vi "Module Loop.vi"(8 "error in (no error)":errorcluster, 11 "DAQmxDO in":refnum<class "DAQmxDO.lvclass">) -> (0 "error out":errorcluster, 3 "DAQmxDO out":refnum<class "DAQmxDO.lvclass">)   [LabVIEW 2023, in "VolatusDAQ.lvlib" / "DAQmxDO.lvclass"]
uses:
  DAQmxDO.lvclass
  DAQmxDO.lvclass/DAQmxDO.ctl
  Volatus/Module/Module.lvclass
  lv-vecto/Vecto/Group DBL/Group DBL.lvclass
  VolatusData/Scaling/Scaling.lvclass
  lv-vecto/Vecto/Group/Group.lvclass
  lv-vecto/Vecto/Vecto.lvlib
  <vilib>/DAQmx/write.llb/DAQmx Write (Digital 1D Bool NChan 1Samp 1Line).vi
  C:/dev/volatus/mts-volatus-super/libs/lv-volatus/Volatus/Module/Module.lvclass
  C:/dev/volatus/mts-volatus-super/libs/lv-volatus/VolatusDAQ/DAQmxDO/DAQmxDO.lvclass
  C:/dev/volatus/mts-volatus-super/libs/lv-vecto/Vecto/Group/Group.lvclass
  C:/dev/volatus/mts-volatus-super/libs/lv-vecto/Vecto/Group DBL/Group DBL.lvclass
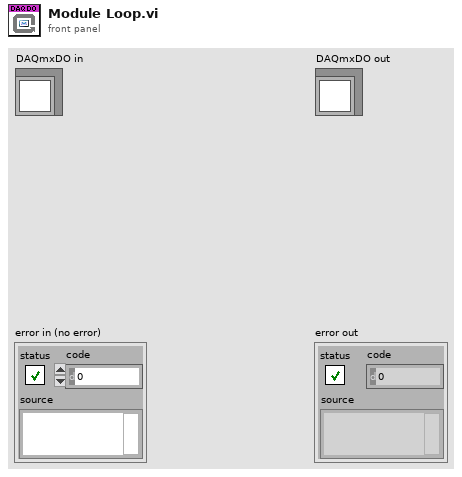
[diagram p1: front panel]
types:
  T1 = enum32{"Invalid", "Standard", "Closed", "Hidden", "Minimized", "Maximized"}
  T2 = typedef "CmdDigitalMultiple.lvlib/Data.ctl" = cluster{"values":T3[]}
  T3 = typedef "CmdDigital.lvlib/Data.ctl" = cluster{"channel":string, "value":bool}
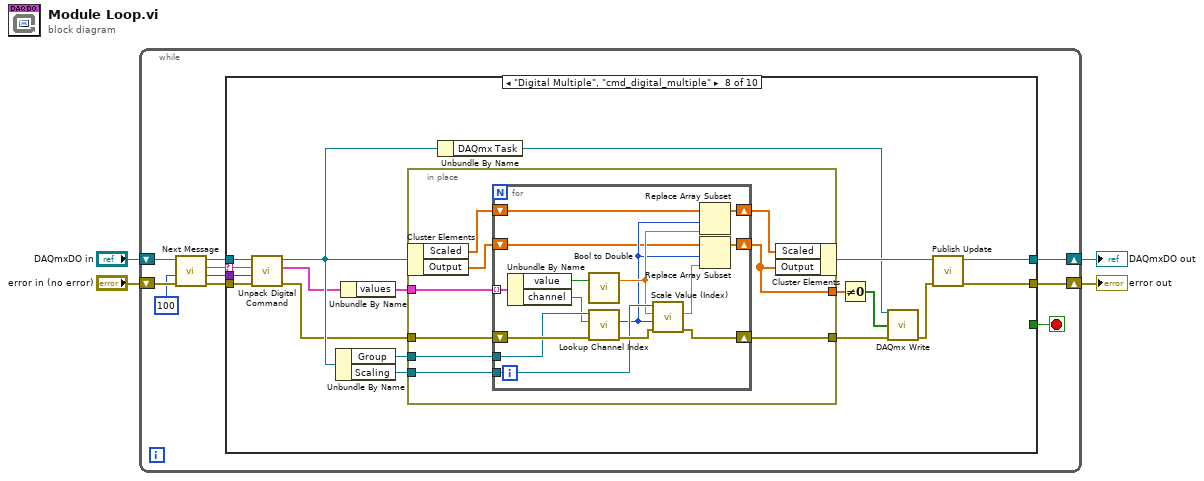
[diagram p0: block diagram]
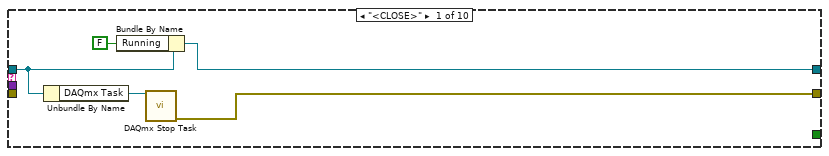
[diagram p2: hidden frame]
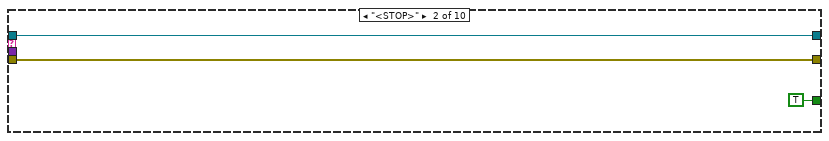
[diagram p3: hidden frame]
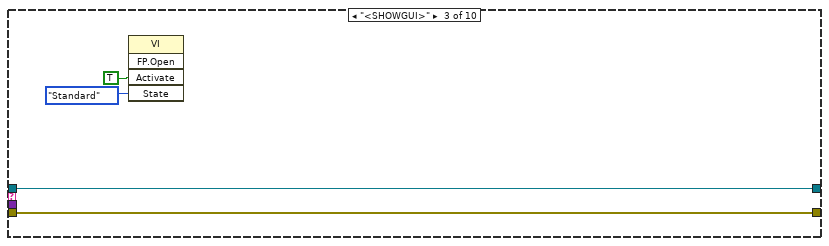
[diagram p4: hidden frame]
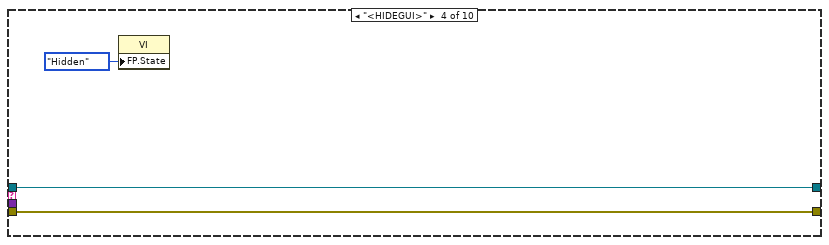
[diagram p5: hidden frame]
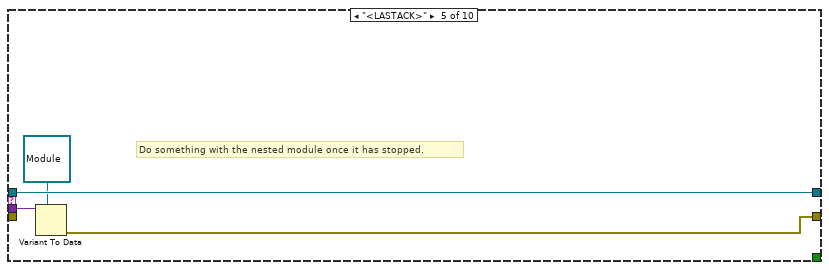
[diagram p6: hidden frame]
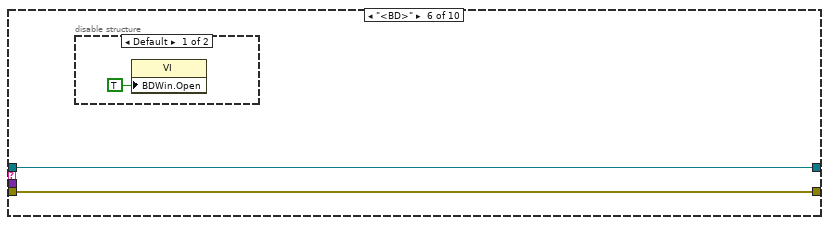
[diagram p7: hidden frame]
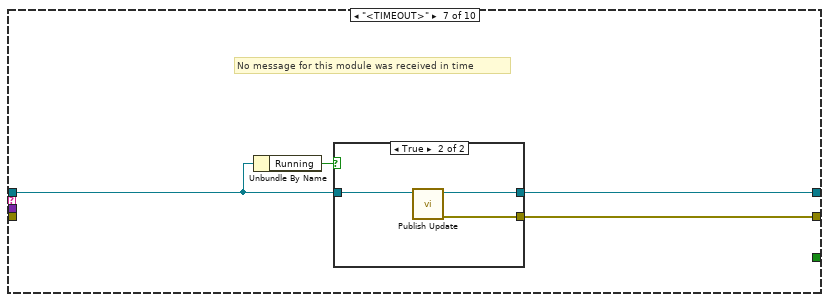
[diagram p9: hidden frame]
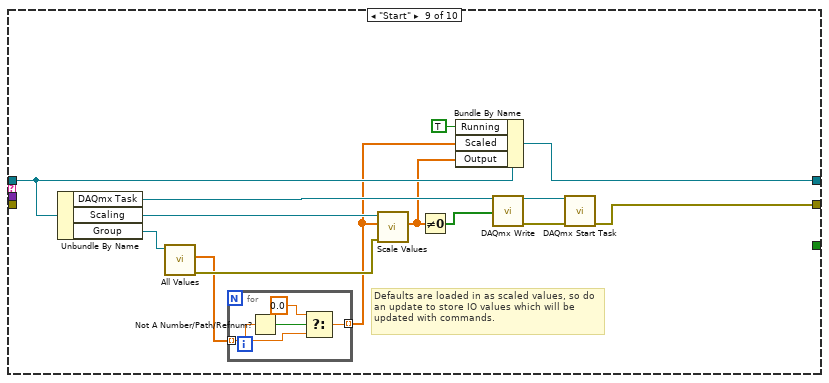
[diagram p11: hidden frame]
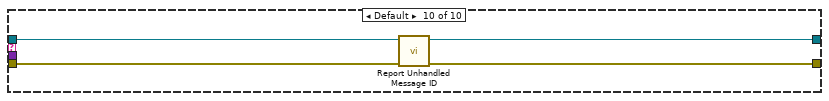
[diagram p12: hidden frame]
diagram:
  n1 = while {
    shift-right: [w9] -> w2
    shift-left: "DAQmxDO in" -> [w14]
    shift-right: [w8] -> w1
    shift-left: "error in (no error)" -> [w13]
    stop <- w7 stop-if-true
    n2 = call "Next Message.vi"("error in (no error)"=w13, "Timeout/Period ms (-1)"=100 ("Timeout ms (-1)"), "Module in"=w14) -> ("error out"=w12:errorcluster, "Data"=w6:variant, "ID"=w11:string, "Module out"=w10:refnum<class "DAQmxDO.lvclass">)  [unwired: 5 in]
    n3 = case shown="\"Digital Multiple\", \"cmd_digital_multiple\"" w11 {
      selector: w11 -> [_ _ _ _ _ _ _ w48 _ _]
      tunnel: w12 -> [_ w21 w25 w28 _ w34 _ w50 _ w108]
      tunnel: w10 -> [w18 w22 w26 w29 w33 w35 w38 w51 w94 w106]
      tunnel: [w16 w22 w26 w29 w33 w35 w39 w52 w90 w105] -> w9
      tunnel: [w17 w21 w25 w28 w30 w34 w40 w53 w93 w107] -> w8
      tunnel: [_ TRUE _ _ _ _ _ _ _ _] -> w7
      tunnel: w6 -> [_ _ _ _ w32 _ _ w49 _ _]
      frame "<CLOSE>" {
        n4 = Unbundle By Name(w18) -> ("DAQmx Task"=w19:refnum<k21>)
        n5 = Bundle By Name(cluster=w18, "Running"=FALSE) -> (w16:refnum<class "DAQmxDO.lvclass">)
        n6 = call <vilib>:"DAQmx Stop Task.vi"("task/channels in"=w19) -> ("error out"=w17:errorcluster)  [unwired: 13 in, 1 out]
      }
      frame "<STOP>" {
      }
      frame "<SHOWGUI>" {
        n7 = invoke class="VI" method="FP.Open"("Activate"=TRUE ("Activate?"), "State"=T1."Standard") -> ()  [unwired: 3 in, 5 out]
      }
      frame "<HIDEGUI>" {
        n8 = property class="VI"("FP.State"=T1."Hidden" ("Front Panel Window:State")) -> ()  [unwired: 2 in, 2 out]
      }
      frame "<LASTACK>" {
        # "Do something with the nested module once it has stopped."
        n9 = Variant To Data(type=refnum<class "Module.lvclass"> refnum ("Volatus:Module"), Variant=w32) -> (error out=w30:errorcluster)  [unwired: 1 in, 1 out]
      }
      frame "<BD>" {
        n10 = disable-structure shown="Default" {
          frame condition #0 (active) {
            n11 = property class="VI"("BDWin.Open"=TRUE ("Block Diagram Window:Open")) -> ()  [unwired: 2 in, 2 out]
          }
          frame condition #1 {
          }
        }
      }
      frame "<TIMEOUT>" {
        # "No message for this module was received in time"
        n12 = Unbundle By Name(w38) -> ("Running"=w37:bool)
        n13 = case shown="True" w37 {
          tunnel: [_ w42] -> w40
          tunnel: [w41 w43] -> w39
          tunnel: w38 -> [w41 w44]
          frame False {
          }
          frame True {
            n14 = call "Publish Update.vi"("DAQmxDO in"=w44) -> ("error out"=w42:errorcluster, "DAQmxDO out"=w43:refnum<class "DAQmxDO.lvclass">)  [unwired: 9 in]
          }
        }
      }
      frame "Digital Multiple", "cmd_digital_multiple" {
        n15 = call "Unpack Digital Command.vi"("error in (no error)"=w50, "Data"=w49, "Type"=w48, "Module in"=w51) -> ("error out"=w45:errorcluster, "CmdDigitalMultiple"=w46:T2, "Module out"=w47:refnum<class "DAQmxDO.lvclass">)  [unwired: 3 in, 2 out]
        n16 = Unbundle By Name(w47) -> ("Group"=w61:refnum<class "Group DBL.lvclass">, "Scaling"=w60:refnum<class "Scaling.lvclass">)
        n17 = Unbundle By Name(w46) -> ("values"=w54:T3[])
        n18 = in-place {
          in-place-border: [w71] -> w62
          in-place-border: w61 -> [w70]
          in-place-border: w60 -> [w69]
          in-place-border: w54 -> [w68]
          in-place-border: w45 -> [w67]
          in-place-border: [w63] -> w58
          n19 = in-place-cluster #1(w47) -> ("Scaled"=w66:dbl[], "Output"=w65:dbl[])
          n20 = for {
            tunnel: w69 -> [w83]
            shift-right: [w79] -> w71
            shift-left: w67 -> [w85]
            tunnel: w68 -> [w82] mode=indexing
            tunnel: w70 -> [w84]
            shift-right: [w75] -> w63
            shift-left: w65 -> [w73]
            shift-right: [w74] -> w64
            shift-left: w66 -> [w72]
            n21 = Unbundle By Name(w82) -> ("value"=w81:bool, "channel"=w80:string)
            n22 = call "Bool to Double.vi"("Bool"=w81) -> ("Double"=w78:dbl)  [unwired: 2 in]
            n23 = call "Lookup Channel Index.vi"("error in (no error)"=w85, "Channel Name"=w80, "Group in"=w84) -> ("error out"=w86:errorcluster, "Index"=w76:i32)  [unwired: 6 in, 1 out]
            n24 = call "Scale Value (Index).vi"("error in (no error)"=w86, "Index"=w76, "Value"=w78, "VolatusScaling in"=w83) -> ("error out"=w79:errorcluster, "Scaled Value"=w77:dbl)  [unwired: 5 in, 1 out]
            n25 = Replace Array Subset(array=w72, new element=w78, index=w76) -> (w74:dbl[])
            n26 = Replace Array Subset(array=w73, new element=w77, index=w76) -> (w75:dbl[])
          }
          n27 = in-place-cluster #1("Scaled"=w64, "Output"=w63) -> (w59:refnum<class "DAQmxDO.lvclass">)
        }
        n28 = Unbundle By Name(w47) -> ("DAQmx Task"=w55:refnum<k21>)
        n29 = Not Equal To 0?(x=w58) -> (x != 0?=w57:bool[])
        n30 = call-poly <vilib>:"DAQmx Write.vi"("task/channels in"=w55, "data"=w57, "error in"=w62) -> ("error out"=w56:errorcluster)  [unwired: 10 in, 2 out]
        n31 = call "Publish Update.vi"("error in (no error)"=w56, "DAQmxDO in"=w59) -> ("error out"=w53:errorcluster, "DAQmxDO out"=w52:refnum<class "DAQmxDO.lvclass">)  [unwired: 8 in]
      }
      frame "Start" {
        # "Defaults are loaded in as scaled values, so do an update to store IO values which will be updated with commands."
        n32 = Unbundle By Name(w94) -> ("DAQmx Task"=w97:refnum<k21>, "Scaling"=w98:refnum<class "Scaling.lvclass">, "Group"=w99:refnum<class "Group DBL.lvclass">)
        n33 = call "All Values.vi"("Group in"=w99) -> ("error out"=w100:errorcluster, "Scaled"=w91:dbl[])  [unwired: 6 in, 3 out]
        n34 = for {
          tunnel: w91 -> [w103] mode=indexing
          tunnel: [w101] -> w89 mode=indexing
          n35 = Not A Number/Path/Refnum?(number/path/refnum=w103) -> (NaN/Path/Refnum?=w104:bool)
          n36 = Select(t=0.0, s=w104, f=w103) -> (s? t:f=w101:dbl)
        }
        n37 = call "Scale Values.vi"("error in (no error)"=w100, "Values"=w89, "VolatusScaling in"=w98) -> ("Scaled Values"=w88:dbl[])  [unwired: 6 in, 2 out]
        n38 = Not Equal To 0?(x=w88) -> (x != 0?=w92:bool[])
        n39 = Bundle By Name(cluster=w94, "Running"=TRUE, "Scaled"=w89, "Output"=w88) -> (w90:refnum<class "DAQmxDO.lvclass">)
        n40 = call-poly <vilib>:"DAQmx Write.vi"("task/channels in"=w97, "data"=w92) -> ("task out"=w96:refnum<k21>, "error out"=w95:errorcluster)  [unwired: 11 in, 1 out]
        n41 = call <vilib>:"DAQmx Start Task.vi"("task/channels in"=w96, "error in"=w95) -> ("error out"=w93:errorcluster)  [unwired: 12 in, 1 out]
      }
      frame Default {
        n42 = call "Report Unhandled Message ID.vi"("error in (no error)"=w108, "Module in"=w106) -> ("error out"=w107:errorcluster, "Module out"=w105:refnum<class "DAQmxDO.lvclass">)  [unwired: 8 in]
      }
    }
  }
  "error out" <- w1
  "DAQmxDO out" <- w2
